vi "test Multiple Clients.vi"(8 "error in (no error)":errorcluster, 11 "TestCase in":refnum<class "test Multiple Clients.lvclass">) -> (0 "error out":errorcluster, 3 "TestCase out":refnum<class "test Multiple Clients.lvclass">)   [LabVIEW 2013, in "test Multiple Clients.lvclass"]
uses:
  test Multiple Clients.lvclass
  dotNET SSL Socket/dotNET SSL Listener/dotNET Listener.lvclass
  dotNET SSL Socket/dotNET TCP Socket/dotNET TCP Socket.lvclass
  <vilib>/MediaMongrels Ltd/WebSockets/Sockets/Socket/Socket.lvclass
  <vilib>/addons/_JKI Toolkits/VI Tester/TestCase.llb/TestCase.lvclass
panel:
  out "Sent":string[](array[string])
  out "Received by Server":string[](array[string])
  out "Returned":string[](array[string])
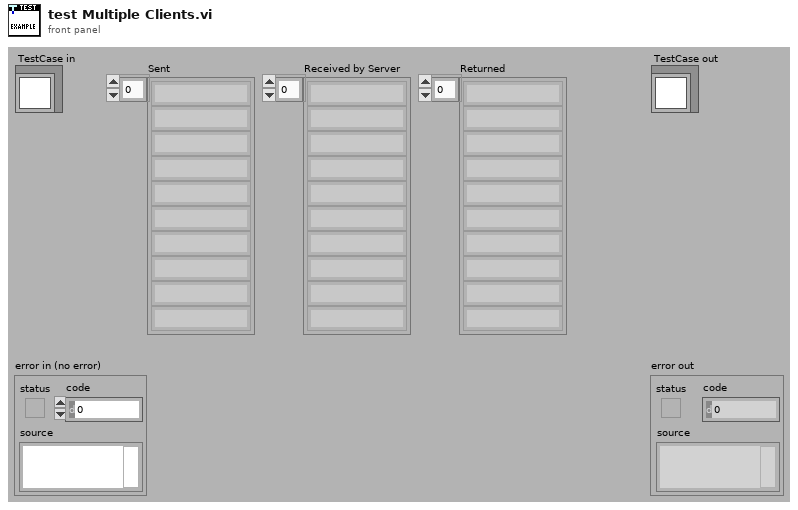
[diagram p1: front panel]
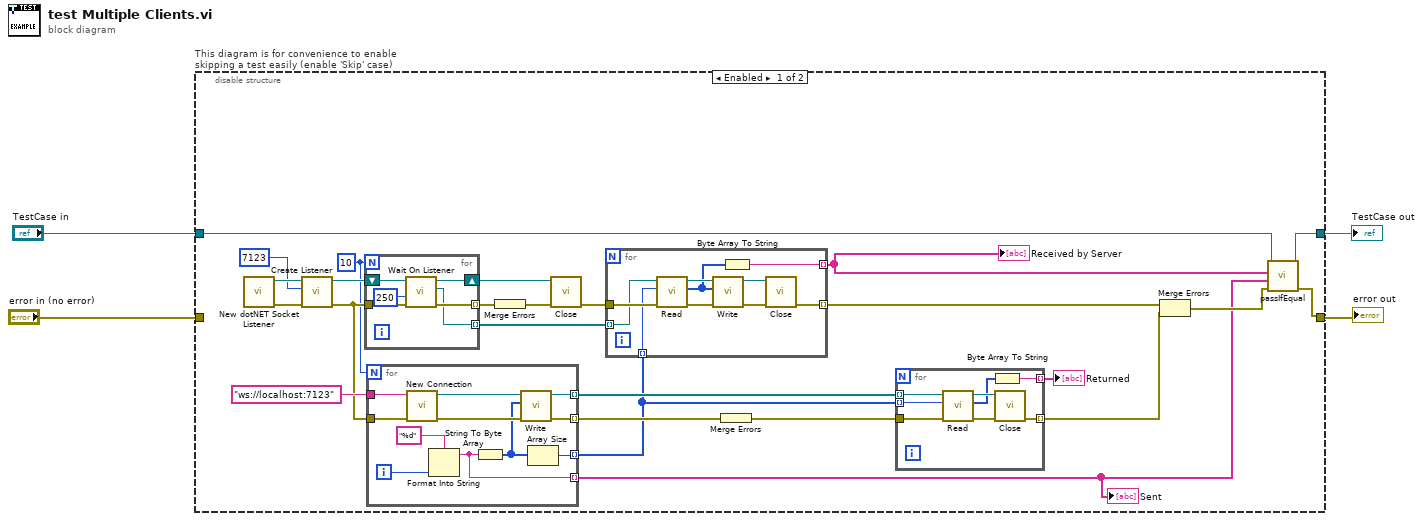
[diagram p0: block diagram]
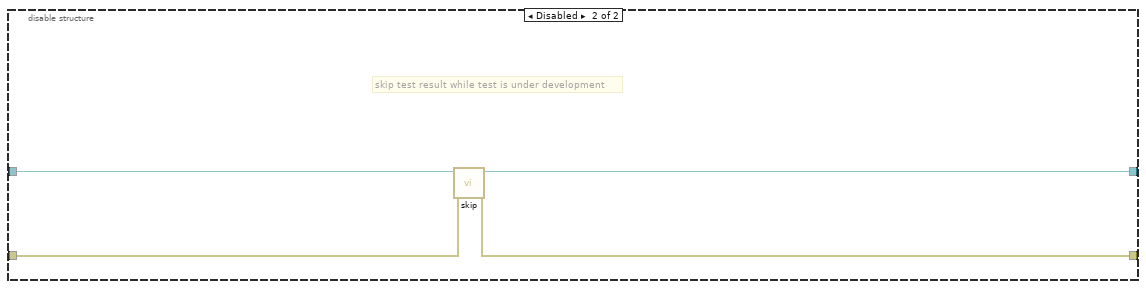
[diagram p2: hidden frame]
diagram:
  n1 = disable-structure "This diagram is for convenience to enable skipping a test easily (enable 'Skip' case)" shown="Enabled" {
    disable-tunnel: "TestCase in" -> [w29 w68]
    disable-tunnel: [w28 w66] -> w1
    disable-tunnel: [w27 w67] -> w3
    disable-tunnel: "error in (no error)" -> [_ w65]
    frame Enabled {
      w14 = 10
      n2 = call "New dotNET Socket Listener.vi"() -> ("error out"=w26:errorcluster, "dotNET Listener out"=w25:refnum<class "dotNET Listener.lvclass">)  [unwired: 10 in]
      n3 = call-dynamic "Create Listener.vi"("error in (no error)"=w26, "Port"=u16 7123, "dotNET Listener in"=w25) -> ("error out"=w21:errorcluster, "dotNET Listener out"=w24:refnum<class "dotNET Listener.lvclass">)  [unwired: 7 in]
      n4 = for {
        N: w14 -> [_]
        tunnel: w21 -> [w63]
        shift-right: [w61] -> w19
        shift-left: w24 -> [w64]
        tunnel: [w62] -> w20 mode=indexing
        tunnel: [w60] -> w17 mode=indexing
        n5 = call-dynamic "Wait On Listener.vi"("error in (no error)"=w63, "timeout ms (5000)"=250, "dotNET Listener in"=w64) -> ("error out"=w62:errorcluster, "Socket out"=w60:refnum<class "Socket.lvclass">, "dotNET Listener out"=w61:refnum<class "dotNET Listener.lvclass">)  [unwired: 6 in]
      }
      n6 = for {
        N: w14 -> [_]
        tunnel: "ws://localhost:7123" ("Hostname / URL") -> [w58]
        tunnel: w21 -> [w57]
        tunnel: [w51] -> w7 mode=indexing
        tunnel: [w50] -> w5 mode=indexing
        tunnel: [w49] -> w12 mode=indexing
        tunnel: [w48] -> w11 mode=indexing
        i -> [w54]
        n7 = call "New Connection.vi"("error in (no error)"=w57, "Hostname / URL"=w58) -> ("error out"=w56:errorcluster, "dotNET TCP Socket out"=w55:refnum<class "dotNET TCP Socket.lvclass">)  [unwired: 8 in]
        n8 = Format Into String(format string="%d", w54) -> (resulting string=w50:string)  [unwired: 2 in, 1 out]
        n9 = String To Byte Array(string=w50) -> (unsigned byte array=w52:u8[])
        n10 = call-dynamic "Write.vi"("error in (no error)"=w56, "Bytes to write"=w52, "dotNET TCP Socket in"=w55) -> ("error out"=w48:errorcluster, "dotNET TCP Socket out"=w49:refnum<class "dotNET TCP Socket.lvclass">)  [unwired: 6 in, 1 out]
        n11 = Array Size(array=w52) -> (size(s)=w51:i32)
      }
      "Sent" <- w5
      n12 = Merge Errors(w20) -> (w18:errorcluster)
      n13 = call-dynamic "Close.vi"("error in (no error)"=w18, "dotNET Listener in"=w19) -> ("error out"=w16:errorcluster)  [unwired: 9 in]
      n14 = for {
        tunnel: w17 -> [w46] mode=indexing
        tunnel: w16 -> [w47]
        tunnel: w7 -> [w45] mode=indexing
        tunnel: [w44] -> w15 mode=indexing
        tunnel: [w38] -> w13 mode=indexing
        n15 = call-dynamic "Read.vi"("error in (no error)"=w47, "# bytes to read"=w45, "Socket in"=w46) -> ("error out"=w42:errorcluster, "Read Bytes"=w39:u8[], "Socket out"=w43:refnum<class "Socket.lvclass">)  [unwired: 6 in]
        n16 = call-dynamic "Write.vi"("error in (no error)"=w42, "Bytes to write"=w39, "Socket in"=w43) -> ("error out"=w41:errorcluster, "Socket out"=w40:refnum<class "Socket.lvclass">)  [unwired: 6 in, 1 out]
        n17 = Byte Array To String(unsigned byte array=w39) -> (string=w44:string)
        n18 = call-dynamic "Close.vi"("error in (no error)"=w41, "Socket in"=w40) -> ("error out"=w38:errorcluster)  [unwired: 9 in]
      }
      "Received by Server" <- w15
      n19 = Merge Errors(w11) -> (w10:errorcluster)
      n20 = for {
        tunnel: w12 -> [w37] mode=indexing
        tunnel: w10 -> [w36]
        tunnel: [w33] -> w9 mode=indexing
        tunnel: w7 -> [w32] mode=indexing
        tunnel: [w30] -> w6 mode=indexing
        n21 = call-dynamic "Read.vi"("error in (no error)"=w36, "# bytes to read"=w32, "dotNET TCP Socket in"=w37) -> ("error out"=w35:errorcluster, "Read Bytes"=w31:u8[], "dotNET TCP Socket out"=w34:refnum<class "dotNET TCP Socket.lvclass">)  [unwired: 6 in]
        n22 = Byte Array To String(unsigned byte array=w31) -> (string=w30:string)
        n23 = call-dynamic "Close.vi"("error in (no error)"=w35, "dotNET TCP Socket in"=w34) -> ("error out"=w33:errorcluster)  [unwired: 9 in]
      }
      "Returned" <- w6
      n24 = Merge Errors(w13, w9) -> (w8:errorcluster)
      n25 = call-dynamic "passIfEqual.vi"("error in (no error)"=w8, "y"=w5, "x"=w15, "TestCase in"=w29) -> ("error out"=w27:errorcluster, "TestCase out"=w28:refnum<class "test Multiple Clients.lvclass">)  [unwired: 6 in]
    }
    frame Disabled {
      # "skip test result while test is under development"
      n26 = call <vilib>:"skip.vi"("error in (no error)"=w65, "TestCase in"=w68) -> ("error out"=w67:errorcluster, "TestCase out"=w66:refnum<class "test Multiple Clients.lvclass">)  [unwired: 8 in]
    }
  }
  "error out" <- w3
  "TestCase out" <- w1
